vi "Hintergrund durchfuehren.vi"() -> ()   [LabVIEW 2020, in "FT-IR.lvlib"]
uses:
  FT-IR.lvlib
  Visualisierungs Elemente/Button.ctl
  Visualisierungs Elemente/Zahlen-Ausgabefeld.ctl
  Visualisierungs Elemente/String - Ausgabefeld.ctl
  Aktionen FT-IR Kalibrieren.ctl
  Stoerungen/Stoerungen Messgeraet/Aktionen Kommunikation Stoerung.ctl
  Schedule Modul/Aktion FGV Testdaten sammeln.ctl
  Funktionstasten/Funktionstasten-Aktion.ctl
  Funktionstasten/Zustaende.ctl
  Messdaten/Aktionen FGV Messdaten.ctl
  FGV FT-IR Gasliste Aktionen.ctl
  Funktionstasten/Freigabe Aktionen.ctl
  SysLog/SysLog Interface.ctl
  Aktionen Zeitstempel speichern.ctl
  FGV FT-IR Aktionen.ctl
  ReadLabFile/Aktionen Lab File.ctl
  Allgemein/allgemeine Sub-VIs.lvlib
  Funktionstasten/Funktionstasten.lvlib
  Messdaten/Messdaten.lvlib
  Stoerungen/Stoerungen.lvlib
  ReadLabFile/Read Lab File.lvlib
  Sprachverwaltung/Sprachverwaltung.lvlib
  SysLog/SysLog.lvlib
  Schedule Modul/Schedule Modul.lvlib
panel:
  out "Konzentration CO2":T1 format="%.2f"
  out "Status":T2
  out "Konzentration H2O":T1 format="%.2f"
  in  "STARTEN":T3
  in  "ABBRECHEN":T3 caption="Abbrechen"
  # "FT-IR Hintergrund"
  # "H2O:"
  # "CO2:"
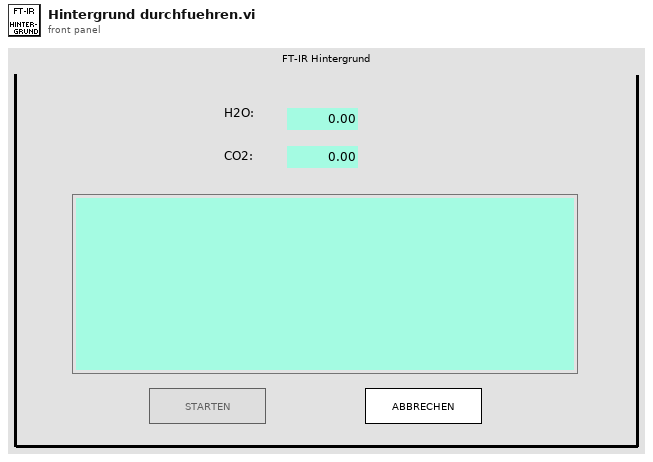
[diagram p1: front panel]
types:
  T1 = typedef "Zahlen-Ausgabefeld.ctl" = sgl
  T2 = typedef "String - Ausgabefeld.ctl" = string
  T3 = typedef "Button.ctl" = bool
  T4 = typedef "Funktionstasten.lvlib/Zustaende.ctl" = enum16{"Standby", "Pause", "Eco", "Messen", "Kalibrieren", "Spülen Filter", "Spülen Leitung", "Umgebungsluft", "0-Gas", "Cal-Gas", "CG zu PNS", "-------------", "Init 1", "Init 2", "Init 3", "Init 4", "Messen vorbereiten", "Messen durchführen", "Exit"}
  T5 = typedef "Funktionstasten.lvlib/Funktionstasten-Aktion.ctl" = enum16{"Initialisieren", "Zustand setzen", "Taste gedrückt", "Fehler speichern", "Lesen", "Manuell", "Remote", "Bitparallel", "Samplepoint", "Zeit Prüfen", "reset Umschalten"}
  T6 = typedef "Stoerungen.lvlib/Aktionen Kommunikation Stoerung.ctl" = enum16{"lesen", "init", "FT-IR Komm", "FT-IR Betriebsart", "FT-IR Hintergrund", "cRIO Komm", "PNS Komm", "Dichtheitstest", "Life Bit", "FTIR Komm AK", "PMA Komm", "FID Komm", "PMA Cal", "FID Ch4 Cal", "FID THC Cal", "Cal Timeout", "VFS 1 Komm", "VFS 2 Komm", "VFS 3 Komm", "VFS 4 Komm", "TRE 08 Komm", "CG-Test vorzeitig", "CG-Test Span 1", "CG-Test Span 2", "CG-Test Span 3", "CG-Test Messgas", "CG-Test löschen", "Test", "Amium AK", "AK Recept konfig", "AK Name konfig", "AK EKFG konfig"}
  T7 = typedef "FT-IR.lvlib/Aktionen FT-IR Kalibrieren.ctl" = enum16{"Initialisieren", "Anstehende Störung", "CO2, H2O - Vergleichen", "Hintergrund starten", "Hintergrund", "Hintergrund Abgeschlossen", "Fertig", "Beenden"}
  T8 = typedef "Funktionstasten.lvlib/Freigabe Aktionen.ctl" = enum16{"prüfen", "Freigabe?", "lesen"}
  T9 = enum8{"Enabled", "Disabled", "Disabled and Grayed Out"}
  T10 = typedef "FT-IR.lvlib/FGV FT-IR Gasliste Aktionen.ctl" = enum16{"lesen", "Gasliste FT-IR", "Gasliste ausgelesen", "laden", "speichern", "löschen"}
  T11 = typedef "Messdaten.lvlib/Aktionen FGV Messdaten.ctl" = enum16{"lesen", "schreiben", "löschen", "Mittelwerte", "Komponente"}
  T12 = typedef "Schedule Modul.lvlib/Aktion FGV Testdaten sammeln.ctl" = enum16{"lesen", "Dichtheitstest", "CalGasTest", "T90", "Kalibrieren", "init", "Kalender Daten"}
  T13 = typedef "Stoerungen.lvlib/Stoerungen Messgeraete.ctl" = cluster{"FT-IR Komm":bool, "FT-IR Betriebsart":bool, "FT-IR Hintergrundscan":bool, "Dichtheitstest":bool, "cRIO Komm":bool, "PNS Komm":bool, "Life Bit":bool, "FT-IR AK Komm":bool, "PMA Komm":bool, "FID Komm":bool, "PMA Cal":bool, "FID CH4 Cal":bool, "FID THC Cal":bool, "Cal Timeout":bool, "VFS 1 Komm":bool, "VFS 2 Komm":bool, "VFS 3 Komm":bool, "VFS 4 Komm":bool, "TRE 08 Komm":bool, "CG-Test":bool, "CG-Test 1":bool, "CG-Test 2":bool, "CG-Test 3":bool, "Messgas - Eingang":bool, "Amium AK Komm":bool, "AK Rezept nicht konfiguriert ":bool, "AK Name nicht konfiguriert":bool, "AK EKFG nicht konfiguriert":bool}
  T14 = typedef "Schedule Modul.lvlib/Ergebnis Kalibrieren.ctl" = cluster{"Fehler":bool, "CO2 H2O vergleich":bool}
  T15 = typedef "SysLog.lvlib/SysLog Interface.ctl" = cluster{"FehlermeldungsCode":i32, "ErfolgsmeldungsCode":i32, "ParameterListenString":string, "Anzeige":bool, "SysLogIcon":enum16{"OK", "Warnung", "Fehler"}, "intern":bool}
  T16 = typedef "FT-IR.lvlib/Aktionen Zeitstempel speichern.ctl" = enum16{"lesen", "Zeitstempel NEU", "laden", "speichern"}
  T17 = typedef "FT-IR.lvlib/Read Lab File.lvlib/Aktionen Lab File.ctl" = enum16{"lesen", "laden"}
  T18 = typedef "FT-IR.lvlib/FGV FT-IR Aktionen.ctl" = enum16{"lesen", "NOG setzen", "NOS setzen", "Initialisieren", "speichern", "ALLES setzen", "FT-IR Spektrum loggen", "Komm Stoppen", "Spektrum LogKonfig"}
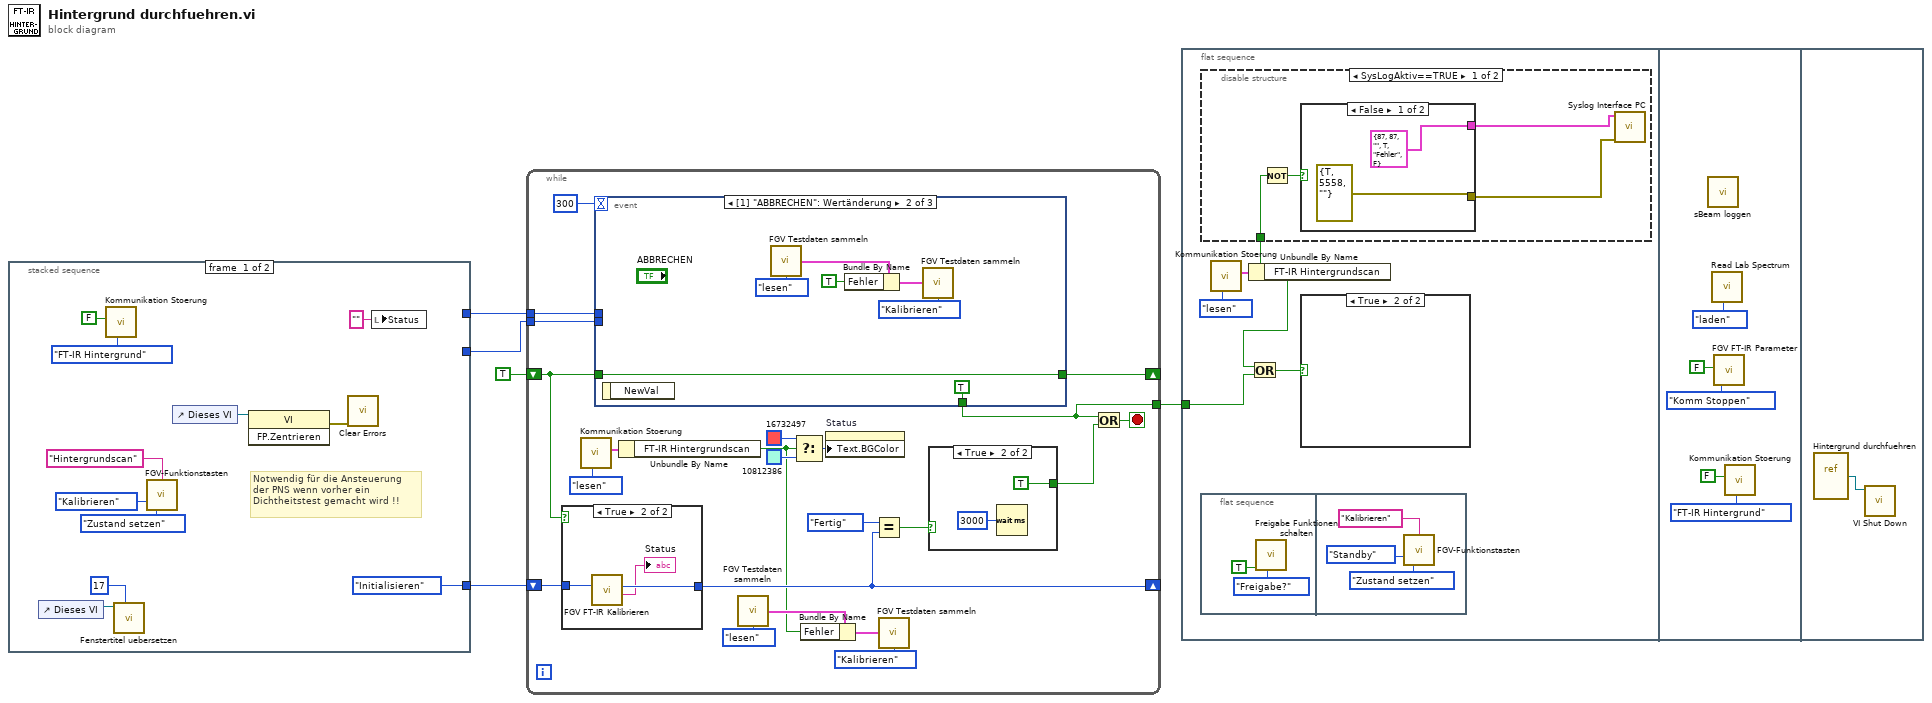
[diagram p0: block diagram]
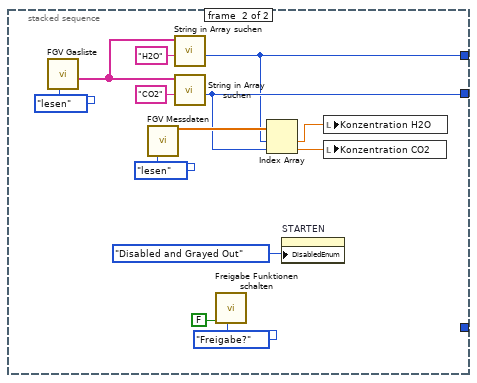
[diagram p2: hidden frame]
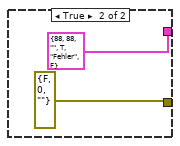
[diagram p3: hidden frame]
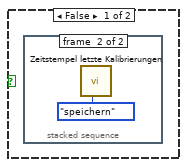
[diagram p5: hidden frame]
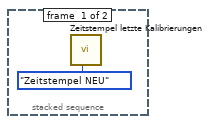
[diagram p6: hidden frame]
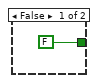
[diagram p7: hidden frame]
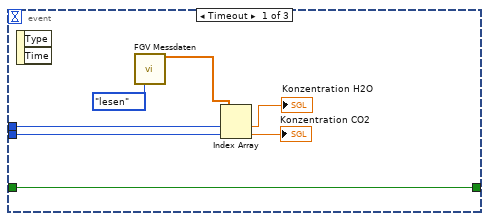
[diagram p9: hidden frame]
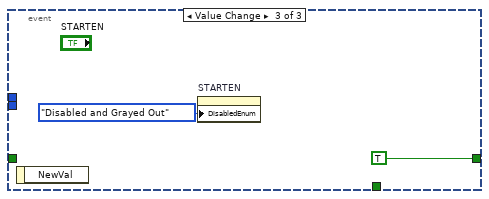
[diagram p10: hidden frame]
diagram:
  n1 = stacked-sequence {
    tunnel: [Aktionen_FT-IR_Kalibrieren."Initialisieren" ("Aktionen FT-IR Kalibrieren") _] -> w4
    tunnel: [_ w21] -> w2
    tunnel: [_ w20] -> w1
    frame #0 {
      # "Notwendig für die Ansteuerung\nder PNS wenn vorher ein \nDichtheitstest gemacht wird !!"
      n2 = control-ref of="Dieses VI"() -> (w12:refnum<vi>)
      n3 = call "Kommunikation Stoerung.vi"("Aktionen"=Aktionen_Kommunikation_Stoerung."FT-IR Hintergrund", "ERROR"=FALSE) -> ()  [unwired: 9 in, 1 out]
      n4 = call "Fenstertitel uebersetzen.vi"("Index (Seite)"=17, "Dieses VI"=w12) -> ()  [unwired: 6 in, 4 out]
      n5 = call "FGV-Funktionstasten.vi"("Herkunft"="Hintergrundscan", "Zustand"=Zustaende."Kalibrieren", "Aktion"=Funktionstasten-Aktion."Zustand setzen") -> ()  [unwired: 5 in, 8 out]
      n6 = control-ref of="Dieses VI"() -> (w10:refnum<vi>)
      n7 = invoke class="VI" method="FP.Zentrieren"(reference=w10) -> (error out=w9:errorcluster)  [unwired: 2 in, 2 out]
      n8 = call <vilib>:"Clear Errors.vi"("error in (no error)"=w9) -> ()  [unwired: 5 in, 2 out]
      n9 = local write "Status"(T2 "" ("Status")) -> ()
    }
    frame #1 {
      n10 = call "FGV Gasliste.vi"("Aktionen"=FGV_FT-IR_Gasliste_Aktionen."lesen") -> ("Aktuelle Gasliste gesamt"=w26:T2[])  [unwired: 8 in, 2 out]
      n11 = call "FGV Messdaten.vi"("Aktionen"=Aktionen_FGV_Messdaten."lesen") -> ("Aktuelle Messwerte"=w27:sgl[])  [unwired: 6 in, 8 out]
      n12 = call "String in Array suchen.vi"("Nach String/Zeichen suchen (-)"="H2O", "String-Array"=w26) -> ("Index"=w20:i32)  [unwired: 7 in, 2 out]
      n13 = call "String in Array suchen.vi"("Nach String/Zeichen suchen (-)"="CO2", "String-Array"=w26) -> ("Index"=w21:i32)  [unwired: 7 in, 2 out]
      n14 = call "Freigabe Funktionen schalten.vi"("Aktionen"=Freigabe_Aktionen."Freigabe?", "Freigabe?"=FALSE) -> ()  [unwired: 7 in, 3 out]
      n15 = Index Array(array=w27, index #1=w20, index #2=w21) -> (element #1=w29:sgl, element #2=w28:sgl)
      n16 = property on="STARTEN" class="Bool."("DisabledEnum"=T9."Disabled and Grayed Out" ("Deaktiviert")) -> ()  [unwired: 2 in, 2 out]
      n17 = local write "Konzentration H2O"(w29) -> ()
      n18 = local write "Konzentration CO2"(w28) -> ()
    }
  }
  n19 = while {
    shift-right: [w50] -> _
    shift-left: TRUE ("STARTEN") -> [w49]
    shift-right: [w45] -> _
    shift-left: w4 -> [w48]
    tunnel: w1 -> [w47]
    tunnel: w2 -> [w46]
    tunnel: [w36] -> w3
    stop <- w43 stop-if-true
    n20 = case shown="True" w49 {
      tunnel: w48 -> [w55 w58]
      tunnel: [w55 w57] -> w45
      frame False {
      }
      frame True {
        n21 = call "FGV FT-IR Kalibrieren.vi"("Aktionen FT-IR Kalibrieren"=w58) -> ("Zustand FT-IR"=→"Status":string, "Aktionen FT-IR Kalibrieren"=w57:T7)  [unwired: 9 in]
      }
    }
    n22 = call "Kommunikation Stoerung.vi"("Aktionen"=Aktionen_Kommunikation_Stoerung."lesen") -> ("Störung Messgerät"=w40:T13)  [unwired: 10 in]
    n23 = event shown="[1] \"ABBRECHEN\": Wertänderung" {
      selector: _ -> [_ _ _]
      dyn-events: _ -> [_ _ _]
      timeout: 300 -> [_ _ _]
      tunnel: [_ TRUE ("ABBRECHEN") _] -> w36
      tunnel: [w65 w71 TRUE ("STARTEN")] -> w50
      tunnel: w49 -> [w65 w71 _]
      tunnel: w47 -> [w64 _ _]
      tunnel: w46 -> [w63 _ _]
      event Timeout {
        n24 = event-data() -> ()  [unwired: 1 in, 2 out]
        n25 = call "FGV Messdaten.vi"("Aktionen"=Aktionen_FGV_Messdaten."lesen") -> ("Aktuelle Messwerte"=w61:sgl[])  [unwired: 6 in, 8 out]
        n26 = Index Array(array=w61, index #1=w64, index #2=w63) -> (element #1=→"Konzentration H2O":sgl, element #2=→"Konzentration CO2":sgl)
      }
      event Value Change {
        n27 = event-data() -> ()  [unwired: 1 in, 1 out]
        n28 = call "FGV Testdaten sammeln.vi"("Aktion"=Aktion_FGV_Testdaten_sammeln."lesen") -> ("Ergebnisse Kalibrieren"=w69:T14)  [unwired: 9 in, 5 out]
        n29 = Bundle By Name(cluster=w69, "Fehler"=TRUE) -> (w70:T14)
        n30 = call "FGV Testdaten sammeln.vi"("Ergebnisse Kalibrieren"=w70, "Aktion"=Aktion_FGV_Testdaten_sammeln."Kalibrieren") -> ()  [unwired: 8 in, 6 out]
      }
      event Value Change {
        n31 = event-data() -> ()  [unwired: 1 in, 1 out]
        n32 = property on="STARTEN" class="Bool."("DisabledEnum"=T9."Disabled and Grayed Out" ("Deaktiviert")) -> ()  [unwired: 2 in, 2 out]
      }
    }
    n33 = Unbundle By Name(w40) -> ("FT-IR Hintergrundscan"=w30:bool)
    n34 = call "FGV Testdaten sammeln.vi"("Aktion"=Aktion_FGV_Testdaten_sammeln."lesen") -> ("Ergebnisse Kalibrieren"=w32:T14)  [unwired: 9 in, 5 out]
    n35 = Select(t=u32 16732497 ("Hintergrund"), s=w30, f=u32 10812386 ("Hintergrund")) -> (s? t:f=w37:u32)
    n36 = Bundle By Name(cluster=w32, "Fehler"=w30) -> (w31:T14)
    n37 = property on="Status" class="Str (strikt)"("Text.BGColor"=w37) -> ()  [unwired: 2 in, 2 out]
    n38 = Equal?(x=Aktionen_FT-IR_Kalibrieren."Fertig", y=w45) -> (x = y?=w35:bool)
    n39 = call "FGV Testdaten sammeln.vi"("Ergebnisse Kalibrieren"=w31, "Aktion"=Aktion_FGV_Testdaten_sammeln."Kalibrieren") -> ()  [unwired: 8 in, 6 out]
    n40 = case shown="True" w35 {
      tunnel: [FALSE TRUE] -> w42
      frame False {
      }
      frame True {
        n41 = Wait (ms)(milliseconds to wait=u32 3000 ("Zu wartende ms")) -> ()  [unwired: 1 out]
      }
    }
    n42 = Or(x=w36, y=w42) -> (x .or. y?=w43:bool)
  }
  n43 = flat-sequence {
    tunnel: w3 -> [w76]
    frame #0 {
      n44 = flat-sequence {
        frame #0 {
          n45 = call "Freigabe Funktionen schalten.vi"("Aktionen"=Freigabe_Aktionen."Freigabe?", "Freigabe?"=TRUE) -> ()  [unwired: 7 in, 3 out]
        }
        frame #1 {
          n46 = call "FGV-Funktionstasten.vi"("Herkunft"="Kalibrieren", "Zustand"=Zustaende."Standby", "Aktion"=Funktionstasten-Aktion."Zustand setzen") -> ()  [unwired: 5 in, 8 out]
        }
      }
      n47 = call "Kommunikation Stoerung.vi"("Aktionen"=Aktionen_Kommunikation_Stoerung."lesen") -> ("Störung Messgerät"=w79:T13)  [unwired: 10 in]
      n48 = Unbundle By Name(w79) -> ("FT-IR Hintergrundscan"=w75:bool)
      n49 = disable-structure shown="SysLogAktiv==TRUE" {
        disable-tunnel: w75 -> [w81 _]
        frame condition #0 (active) {
          n50 = Not(x=w81) -> (.not. x?=w83:bool)
          n51 = case shown="False" w83 {
            tunnel: [errorcluster {"status"=TRUE, "code"=5558, "source"=""} ("Fehler (in)") errorcluster {"status"=FALSE, "code"=0, "source"=""} ("Fehler (in)")] -> w82
            tunnel: [T15 {"FehlermeldungsCode"=87, "ErfolgsmeldungsCode"=87, "ParameterListenString"="", "Anzeige"=TRUE, "SysLogIcon"=enum."Fehler", "intern"=FALSE} ("Cluster (in)") T15 {"FehlermeldungsCode"=88, "ErfolgsmeldungsCode"=88, "ParameterListenString"="", "Anzeige"=TRUE, "SysLogIcon"=enum."Fehler", "intern"=FALSE} ("Cluster (in)")] -> w80
            frame False {
            }
            frame True {
            }
          }
          n52 = call "Syslog Interface PC.vi"("Fehler (in)"=w82, "Cluster (in)"=w80) -> ()  [unwired: 9 in, 1 out]
        }
        frame condition #1 {
        }
      }
      n53 = Or(x=w75, y=w76) -> (x .or. y?=w77:bool)
      n54 = case shown="True" w77 {
        frame False {
          n55 = stacked-sequence {
            frame #0 {
              n56 = call "Zeitstempel letzte Kalibrierungen.vi"("Aktionen"=Aktionen_Zeitstempel_speichern."Zeitstempel NEU") -> ()  [unwired: 10 in, 1 out]
            }
            frame #1 {
              n57 = call "Zeitstempel letzte Kalibrierungen.vi"("Aktionen"=Aktionen_Zeitstempel_speichern."speichern") -> ()  [unwired: 10 in, 1 out]
            }
          }
        }
        frame True {
        }
      }
    }
    frame #1 {
      n58 = call "sBeam loggen.vi"() -> ()  [unwired: 11 in, 1 out]
      n59 = call "Read Lab Spectrum.VI"("Aktionen"=Aktionen_Lab_File."laden") -> ()  [unwired: 7 in, 4 out]
      n60 = call "FGV FT-IR Parameter.vi"("Komm Stoppen"=FALSE, "Aktion"=FGV_FT-IR_Aktionen."Komm Stoppen") -> ()  [unwired: 10 in, 8 out]
      n61 = call "Kommunikation Stoerung.vi"("Aktionen"=Aktionen_Kommunikation_Stoerung."FT-IR Hintergrund", "ERROR"=FALSE) -> ()  [unwired: 9 in, 1 out]
    }
    frame #2 {
      n62 = vi-ref "Hintergrund durchfuehren.vi"() -> (w100:refnum<vi>)
      n63 = call "VI Shut Down.vi"("VI Referenz"=w100) -> ()  [unwired: 11 in]
    }
  }
